vi "TakeSweep.vi"(0 "Session In":refnum<visa-resource-name>="GPIB0::22::INSTR", 7 "error in":errorcluster {"code" format="%.0x"}, 9 "Timeout":u32=5000) -> (20 "Session Out":refnum<visa-resource-name>, 26 "token":dbl, 27 "error out":errorcluster {"code" format="%.0x"})   [LabVIEW 2018]
doc: "Launches the Instrument I/O Assistant, which you can use to communicate with message-based instruments and graphically parse the response. For example you can communicate with an instrument that uses a serial, Ethernet, or GPIB interface."
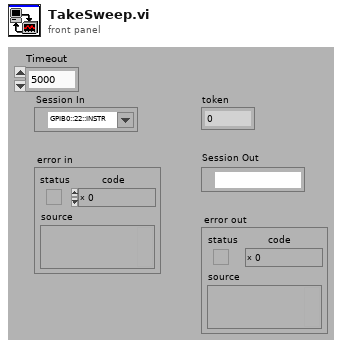
[diagram p1: front panel]
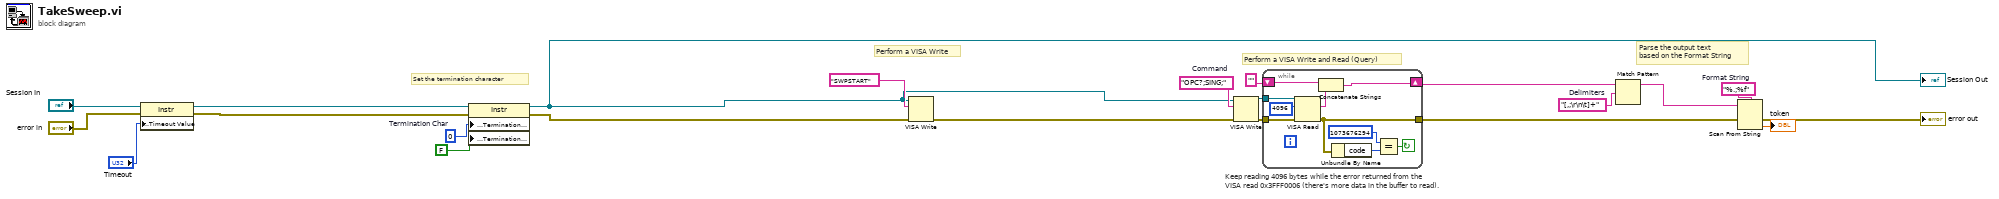
[diagram p0: block diagram]
diagram:
  w2 = "[,;\r\n\t]+"  # Delimiters
  w5 = "%.;%f"  # Format String
  w8 = "OPC?;SING;"  # Command
  w17 = u8 0  # Termination Char
  # "Parse the output text based on the Format String"
  # "Perform a VISA Write and Read (Query)"
  # "Keep reading 4096 bytes while the error returned from the\nVISA read 0x3FFF0006 (there's more data in the buffer to read)."
  # "Perform a VISA Write"
  # "Set the termination character"
  n1 = property class="Instr"(reference="Session In", error in="error in", "General Settings:Timeout Value"="Timeout") -> (reference out=w16:refnum<visa-resource-name>, error out=w19:errorcluster)
  n2 = property class="Instr"(reference=w16, error in=w19, "Message Based Settings:Termination Character"=w17, "Message Based Settings:Termination Character Enable"=FALSE ("enable")) -> (reference out=w1:refnum<visa-resource-name>, error out=w18:errorcluster)
  "Session Out" <- w1
  n3 = VISA Write(VISA resource name=w1, write buffer="SWPSTART" ("StaticText"), error in (no error)=w18) -> (error out=w14:errorcluster)  [unwired: 2 out]
  n4 = VISA Write(VISA resource name=w1, write buffer=w8, error in (no error)=w14) -> (VISA resource name out=w12:refnum<visa-resource-name>, error out=w11:errorcluster)  [unwired: 1 out]
  n5 = while {
    tunnel: w12 -> [w29]
    shift-right: [w23] -> w7
    shift-left: "" -> [w28]
    tunnel: w11 -> [w26]
    tunnel: [w25] -> w10
    stop <- w24 continue-if-true
    n6 = VISA Read(VISA resource name=w29, byte count=u32 4096 ("byte count (0)"), error in (no error)=w26) -> (read buffer=w27:string, error out=w25:errorcluster)  [unwired: 2 out]
    n7 = Concatenate Strings(w28, w27) -> (w23:string)
    n8 = Unbundle By Name(w25) -> ("code"=w31:i32)
    n9 = Equal?(x=1073676294, y=w31) -> (x = y?=w24:bool)
  }
  n10 = Match Pattern(string=w7, regular expression=w2) -> (before substring=w6:string)  [unwired: 1 in, 3 out]
  n11 = Scan From String(format string=w5, input string=w6, error in=w10) -> (error out=→"error out":errorcluster, output 1=→"token":dbl)  [unwired: 2 in, 2 out]
